vi "Update Latest Message Data.vi"(8 "error in (no error)":errorcluster, 10 "Latest Messages":map{string, refnum<class "Debug Data.lvclass">}(c390), 11 "List Seen Processes View Model In":refnum<class "Process Tree View Model.lvclass">) -> (0 "error out":errorcluster, 3 "List Seen Processes View Model Out":refnum<class "Process Tree View Model.lvclass">)   [LabVIEW 2020, in "Process Tree View Model.lvclass"]
uses:
  Process Tree View Model.lvclass
  Debug Data/Debug Data.lvclass
  Process Tree View Model.lvclass/Process Tree View Model.ctl
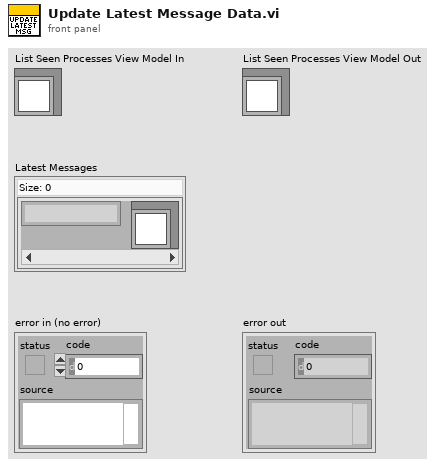
[diagram p1: front panel]
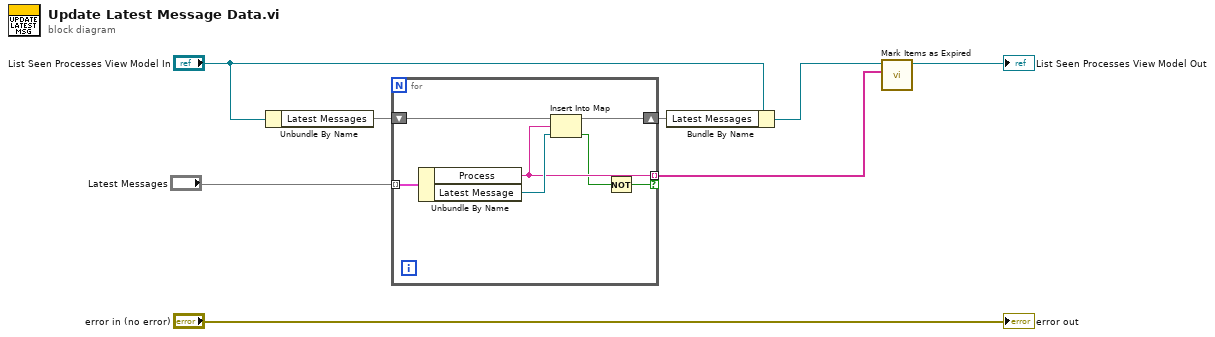
[diagram p0: block diagram]
diagram:
  n1 = Unbundle By Name("List Seen Processes View Model In") -> ("Latest Messages"=w6:map{string, refnum<class "Debug Data.lvclass">})
  n2 = for {
    shift-right: [w12] -> w5
    shift-left: w6 -> [w14]
    tunnel: "Latest Messages" -> [w15] mode=indexing
    tunnel: [w11] -> w2 mode=indexing if=w9
    n3 = Unbundle By Name(w15) -> ("Process"=w11:string, "Latest Message"=w13:refnum<class "Debug Data.lvclass">)
    n4 = Insert Into Map(map in=w14, key=w11, value=w13) -> (map out=w12:map{string, refnum<class "Debug Data.lvclass">}, value unchanged?=w10:bool)  [unwired: 1 out]
    n5 = Not(x=w10) -> (.not. x?=w9:bool)
  }
  n6 = Bundle By Name(cluster="List Seen Processes View Model In", "Latest Messages"=w5) -> (w4:refnum<class "Process Tree View Model.lvclass">)
  n7 = call "Mark Items as Expired.vi"("Expired Tags"=w2, "Process Tree View Model in"=w4) -> ("Process Tree View Model out"=→"List Seen Processes View Model Out":refnum<class "Process Tree View Model.lvclass">)  [unwired: 9 in]
  "error out" <- "error in (no error)"
